vi "Query Plug-In.vi"(8 "error in (no error)":errorcluster, 11 "VISA resource name":refnum<visa-resource-name>) -> (0 "error out":errorcluster, 1 "Plug-In Accessory":u8[](array[numeric]), 2 "Number Of Plug-Ins":u8, 3 "VISA resource name out":refnum<visa-resource-name>)   [LabVIEW 2018, in "Ocean Optics 2000 4000.lvlib"]
doc: "Returns the number of plug-in and also identify the plug-in type."
uses:
  Ocean Optics 2000 4000.lvlib
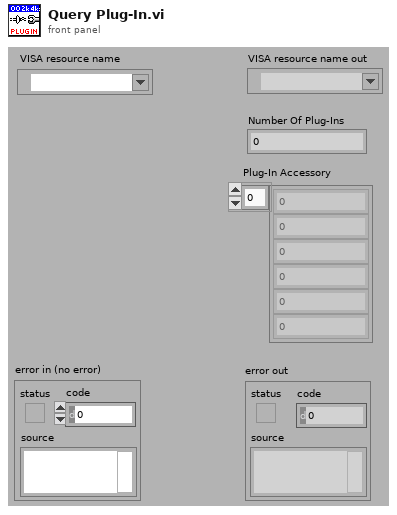
[diagram p1: front panel]
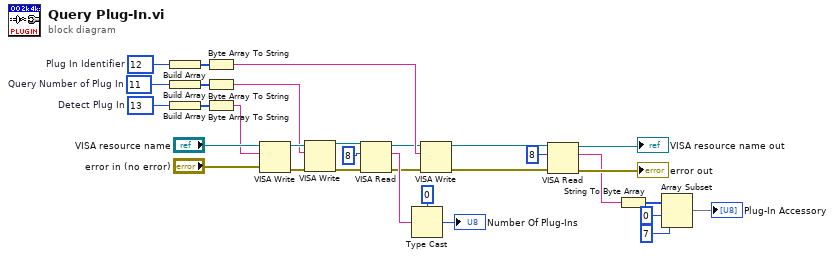
[diagram p0: block diagram]
diagram:
  w17 = u8 12  # Plug In Identifier
  w23 = u8 11  # Query Number of Plug In
  w29 = u8 13  # Detect Plug In
  n1 = Build Array(w17) -> (w16:u8[])
  n2 = Build Array(w23) -> (w24:u8[])
  n3 = Build Array(w29) -> (w28:u8[])
  n4 = Byte Array To String(unsigned byte array=w16) -> (string=w15:string)
  n5 = Byte Array To String(unsigned byte array=w24) -> (string=w22:string)
  n6 = Byte Array To String(unsigned byte array=w28) -> (string=w27:string)
  n7 = VISA Write(VISA resource name="VISA resource name", write buffer=w27, error in (no error)="error in (no error)") -> (VISA resource name out=w25:refnum<visa-resource-name>, error out=w26:errorcluster)  [unwired: 1 out]
  n8 = VISA Write(VISA resource name=w25, write buffer=w22, error in (no error)=w26) -> (VISA resource name out=w11:refnum<visa-resource-name>, error out=w10:errorcluster)  [unwired: 1 out]
  n9 = VISA Read(VISA resource name=w11, byte count=u32 8, error in (no error)=w10) -> (VISA resource name out=w9:refnum<visa-resource-name>, read buffer=w19:string, error out=w8:errorcluster)  [unwired: 1 out]
  n10 = Type Cast(type=u8 0, x=w19) -> (*(type *) &x=→"Number Of Plug-Ins":u8)
  n11 = VISA Write(VISA resource name=w9, write buffer=w15, error in (no error)=w8) -> (VISA resource name out=w7:refnum<visa-resource-name>, error out=w6:errorcluster)  [unwired: 1 out]
  n12 = VISA Read(VISA resource name=w7, byte count=u32 8, error in (no error)=w6) -> (VISA resource name out=→"VISA resource name out":refnum<visa-resource-name>, read buffer=w5:string, error out=→"error out":errorcluster)  [unwired: 1 out]
  n13 = String To Byte Array(string=w5) -> (unsigned byte array=w4:u8[])
  n14 = Array Subset(array=w4, index=0, length=7) -> (→"Plug-In Accessory":u8[])
